vi "Main.vi"() -> ()   [LabVIEW 2025]
uses:
  <vilib>/LabVIEW Interface for Arduino/Type Defs/Board Type.ctl
  <vilib>/LabVIEW Interface for Arduino/Type Defs/Connection Type.ctl
  <vilib>/LabVIEW Interface for Arduino/Type Defs/Pin Mode.ctl
  <vilib>/LabVIEW Interface for Arduino/LabVIEW Interface for Arduino.lvlib
panel:
  out "Waveform Chart":dbl(graph)
  out "Light bulb":bool
  in  "Stop":bool
  in  "Switch":bool
  in  "VISA resource":refnum<visa-resource-name>
  # "AUTOMATIC LIGHT SWITCH"
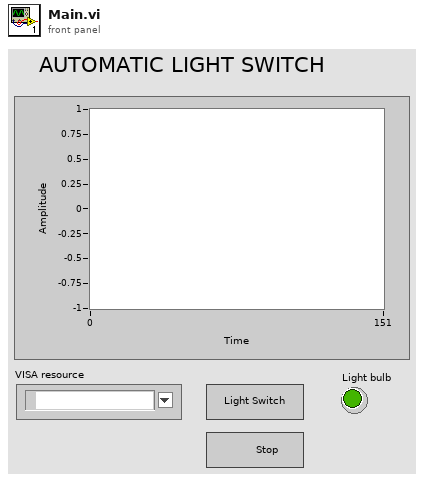
[diagram p1: front panel]
types:
  T1 = typedef "LabVIEW Interface for Arduino.lvlib/Pin Mode.ctl" = enum8{"Input", "Output"}
  T2 = typedef "LabVIEW Interface for Arduino.lvlib/Connection Type.ctl" = enum8{"USB / Serial", "XBEE", "BlueSmirf (Bluetooth)"}
  T3 = typedef "LabVIEW Interface for Arduino.lvlib/Board Type.ctl" = enum16{"Uno", "Dimuelanove w/Atmega 328", "Mega 2560"}
  T4 = typedef "LabVIEW Interface for Arduino.lvlib/Arduino Resource.ctl" = cluster{"VISA resource":refnum<visa-resource-name>, "Board Type":T3, "Connection Type":enum8{"USB / Serial"}, "Bytes Per Packet (15)":u8}
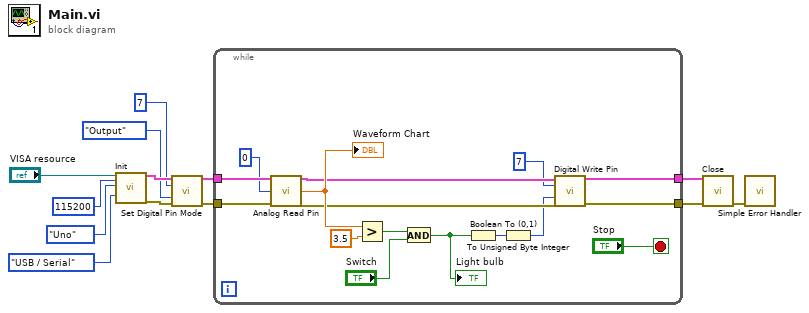
[diagram p0: block diagram]
diagram:
  n1 = call <vilib>:"Init.vi"("VISA resource"="VISA resource", "Baud Rate (115200)"=u32 115200, "Board Type (Uno)"=Board_Type."Uno", "Connection Type (USB/Serial)"=Connection_Type."USB / Serial") -> ("Arduino Resource"=w9:T4, "error out"=w8:errorcluster)  [unwired: 14 in]
  n2 = call <vilib>:"Set Digital Pin Mode.vi"("Arduino Resource"=w9, "Digital I/O Pin"=u8 7 ("Digital I/O Pin (0)"), "Pin Mode (Input)"=Pin_Mode."Output", "error in"=w8) -> ("Arduino Resource"=w5:T4, "error out"=w4:errorcluster)  [unwired: 10 in]
  n3 = while {
    tunnel: w5 -> [w29]
    tunnel: w4 -> [w28]
    tunnel: [w15] -> w3
    tunnel: [w14] -> w2
    stop <- "Stop" stop-if-true
    n4 = call <vilib>:"Analog Read Pin.vi"("Arduino Resource"=w29, "Analog Input Pin (0)"=u8 0, "error in"=w28) -> ("Arduino Resource"=w21:T4, "Voltage"=w26:dbl, "error out"=w20:errorcluster)  [unwired: 10 in]
    "Waveform Chart" <- w26
    n5 = Greater?(x=w26, y=3.5) -> (0:w24:bool)
    n6 = And(x=w24, y="Switch") -> (x .and. y?=w19:bool)
    "Light bulb" <- w19
    n7 = Boolean To (0,1)(Boolean=w19) -> (0, 1=w18:i16)
    n8 = To Unsigned Byte Integer(number=w18) -> (unsigned 8bit integer=w17:u8)
    n9 = call <vilib>:"Digital Write Pin.vi"("Arduino Resource"=w21, "Digital I/O Pin (0)"=u8 7, "Value (0)"=w17, "error in"=w20) -> ("Arduino Resource"=w15:T4, "error out"=w14:errorcluster)  [unwired: 10 in]
  }
  n10 = call <vilib>:"Close.vi"("Arduino Resource"=w3, "error in"=w2) -> ("error out"=w1:errorcluster)  [unwired: 13 in]
  n11 = call <vilib>:"Simple Error Handler.vi"("error in (no error)"=w1) -> ()  [unwired: 4 in, 5 out]
